vi "Get Keys Array.vi"(8 "error in":errorcluster caption="错误输入（无错误）", 11 "Dictionary in":refnum<class "Dictionary.lvclass">) -> (0 "error out":errorcluster caption="错误输出", 2 "Keys Array":string[](array[string]), 3 "Dictionary out":refnum<class "Dictionary.lvclass">)   [LabVIEW 2012, in "Dictionary.lvclass"]
uses:
  Dictionary.lvclass
  Dictionary.lvclass/Dictionary.ctl
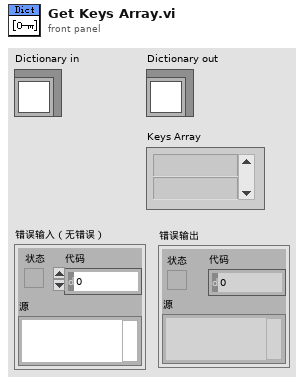
[diagram p1: front panel]
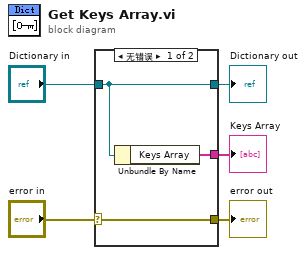
[diagram p0: block diagram]
diagram:
  n1 = case shown="无错误" "error in" {
    selector: "error in" -> [w8 w9]
    tunnel: [w8 w9] -> w4
    tunnel: [w7 w10] -> w2
    tunnel: "Dictionary in" -> [w7 w10]
    tunnel: [w6 _] -> w1
    frame No Error {
      n2 = Unbundle By Name(w7) -> ("Keys Array"=w6:string[])
    }
    frame Error {
    }
  }
  "error out" <- w4
  "Dictionary out" <- w2
  "Keys Array" <- w1
